vi "SubVI_TeleopIntakeWheels_Teleop.vi"(9 "WheelsShootOut":dbl, 10 "WheelsTakeIn":dbl) -> ()   [LabVIEW 2017]
uses:
  <vilib>/Rock Robotics/WPI/ThirdParty/Phoenix-LabVIEW/Motor Controller/Controls/CTRE_Phoenix_MotorControl_ControlMode.ctl
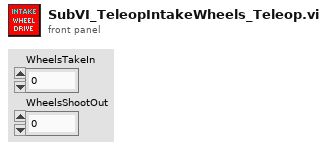
[diagram p1: front panel]
types:
  T1 = typedef "CTRE_Phoenix_MotorControl_ControlMode.ctl" = u16
  T2 = typedef "WPI_MotorControlDeviceRef.ctl" = cluster{"DeviceStatus":errorcluster, "Type":T3, "PWM":cluster{"PWM Channel":T4, "DeadBand":T5}, "CAN":cluster{"Device Number":u8, "SetOutput VI Ref":variant, "GetOutput VI Ref":variant, "Enable VI Ref":variant, "Disable VI Ref":variant, "Data":variant}, "Invert":bool, "DIO PWM":cluster{"PWM \"Enable\" Channel":T4, "DIOChannel":T6, "PWM Rate":dbl}}
  T3 = typedef "WPI_MotorControlType.ctl" = enum16{"PWM", "CAN", "DIO PWM"}
  T4 = typedef "FPGA_DIOPWMChannel.ctl" = enum8{"PWM 0", "PWM 1", "PWM 2", "PWM 3", "PWM 4", "PWM 5", "PWM 6", "PWM 7", "PWM 8", "PWM 9", "PWM MXP 0", "PWM MXP 1", "PWM MXP 2", "PWM MXP 3", "PWM MXP 4", "PWM MXP 5", "PWM MXP 6", "PWM MXP 7", "PWM MXP 8", "PWM MXP 9", "Invalid"}
  T5 = typedef "WPI_PWMDeadband.ctl" = cluster{"Name":string, "maxPositivePwm":i32, "minPositivePwm":i32, "centerPwm":i32, "maxNegativePwm":i32, "minNegativePwm":i32, "angularRange":u16}
  T6 = typedef "FPGA_DIOChannel.ctl" = enum8{"DIO 0", "DIO 1", "DIO 2", "DIO 3", "DIO 4", "DIO 5", "DIO 6", "DIO 7", "DIO 8", "DIO 9", "DIO MXP 0", "DIO MXP 1", "DIO MXP 2", "DIO MXP 3", "DIO MXP 4", "DIO MXP 5", "DIO MXP 6", "DIO MXP 7", "DIO MXP 8", "DIO MXP 9", "DIO MXP 10", "DIO MXP 11", "DIO MXP 12", "DIO MXP 13", "DIO MXP 14", "DIO MXP 15", "SPI Port CS1", "SPI Port CS2", "SPI Port CS3", "SPI Port MISO", "SPI Port MOSI", "Invalid"}
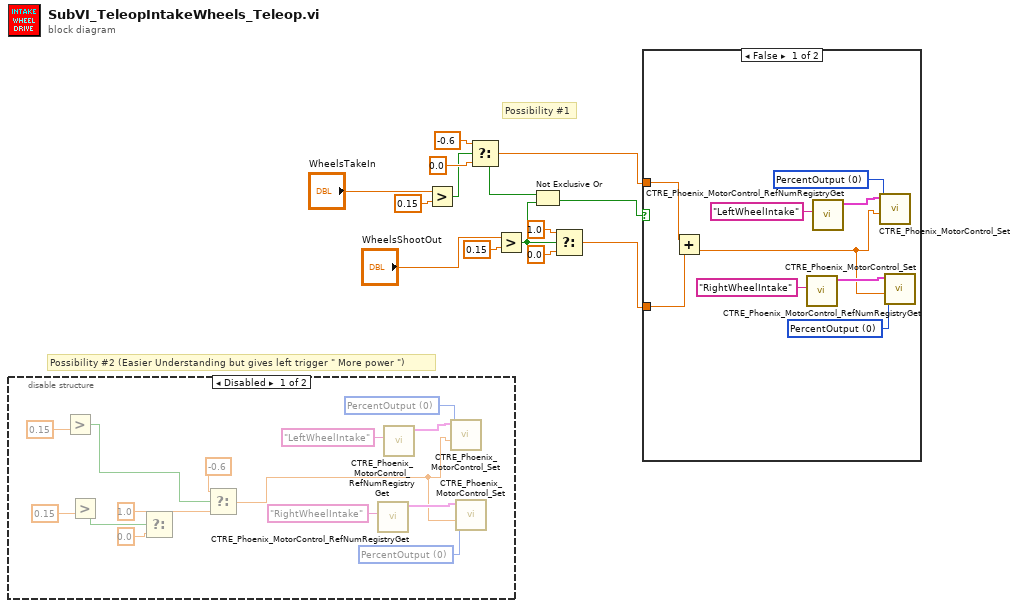
[diagram p0: block diagram]
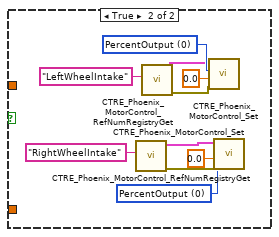
[diagram p3: hidden frame]
diagram:
  # "Possibility #1"
  # "Possibility #2 (Easier Understanding but gives left trigger \" More power \")"
  n1 = disable-structure shown="Disabled" {
    frame Disabled {
      w27 = T1 0 items=["PercentOutput"=0, "Position"=1, "Velocity"=2, "Current"=3, "Follower"=5, "MotionProfile"=6, "MotionMagic"=7, "MotionMagicArc"=8, "MotionProfileArc"=10, "Disabled"=15] ("Control Mode")
      w28 = T1 0 items=["PercentOutput"=0, "Position"=1, "Velocity"=2, "Current"=3, "Follower"=5, "MotionProfile"=6, "MotionMagic"=7, "MotionMagicArc"=8, "MotionProfileArc"=10, "Disabled"=15] ("Control Mode")
      n2 = Greater?(y=0.15) -> (0:w15:bool)  [unwired: 1 in]
      n3 = Greater?(y=0.15) -> (0:w18:bool)  [unwired: 1 in]
      n4 = Select(t=1.0, s=w18, f=0.0) -> (s? t:f=w16:dbl)
      n5 = Select(t=-0.6, s=w15, f=w16) -> (s? t:f=w14:dbl)
      n6 = call <vilib>:"CTRE_Phoenix_MotorControl_RefNumRegistryGet.vi"("refnum name"="RightWheelIntake") -> ("PhoenixMotorControlDevRef"=w25:T2)  [unwired: 9 in, 1 out]
      n7 = call <vilib>:"CTRE_Phoenix_MotorControl_RefNumRegistryGet.vi"("refnum name"="LeftWheelIntake") -> ("PhoenixMotorControlDevRef"=w26:T2)  [unwired: 9 in, 1 out]
      n8 = call <vilib>:"CTRE_Phoenix_MotorControl_Set.vi"("Output"=w14, "Control Mode"=w27, "PhoenixMotorControlDevRef"=w26) -> ()  [unwired: 7 in, 2 out]
      n9 = call <vilib>:"CTRE_Phoenix_MotorControl_Set.vi"("Output"=w14, "Control Mode"=w28, "PhoenixMotorControlDevRef"=w25) -> ()  [unwired: 7 in, 2 out]
    }
    frame Enabled {
    }
  }
  n10 = Greater?(x="WheelsTakeIn", y=0.15) -> (0:w1:bool)
  n11 = Select(t=-0.6, s=w1, f=0.0) -> (s? t:f=w5:dbl)
  n12 = Greater?(x="WheelsShootOut", y=0.15) -> (0:w2:bool)
  n13 = Not Exclusive Or(1:w2, 2:w1) -> (0:w3:bool)
  n14 = Select(t=1.0, s=w2, f=0.0) -> (s? t:f=w4:dbl)
  n15 = case shown="False" w3 {
    tunnel: w5 -> [w31 _]
    tunnel: w4 -> [w30 _]
    frame False {
      w36 = T1 0 items=["PercentOutput"=0, "Position"=1, "Velocity"=2, "Current"=3, "Follower"=5, "MotionProfile"=6, "MotionMagic"=7, "MotionMagicArc"=8, "MotionProfileArc"=10, "Disabled"=15] ("Control Mode")
      w37 = T1 0 items=["PercentOutput"=0, "Position"=1, "Velocity"=2, "Current"=3, "Follower"=5, "MotionProfile"=6, "MotionMagic"=7, "MotionMagicArc"=8, "MotionProfileArc"=10, "Disabled"=15] ("Control Mode")
      n16 = Add(x=w31, y=w30) -> (x+y=w29:dbl)
      n17 = call <vilib>:"CTRE_Phoenix_MotorControl_RefNumRegistryGet.vi"("refnum name"="RightWheelIntake") -> ("PhoenixMotorControlDevRef"=w34:T2)  [unwired: 9 in, 1 out]
      n18 = call <vilib>:"CTRE_Phoenix_MotorControl_RefNumRegistryGet.vi"("refnum name"="LeftWheelIntake") -> ("PhoenixMotorControlDevRef"=w35:T2)  [unwired: 9 in, 1 out]
      n19 = call <vilib>:"CTRE_Phoenix_MotorControl_Set.vi"("Output"=w29, "Control Mode"=w36, "PhoenixMotorControlDevRef"=w35) -> ()  [unwired: 7 in, 2 out]
      n20 = call <vilib>:"CTRE_Phoenix_MotorControl_Set.vi"("Output"=w29, "Control Mode"=w37, "PhoenixMotorControlDevRef"=w34) -> ()  [unwired: 7 in, 2 out]
    }
    frame True {
      w43 = T1 0 items=["PercentOutput"=0, "Position"=1, "Velocity"=2, "Current"=3, "Follower"=5, "MotionProfile"=6, "MotionMagic"=7, "MotionMagicArc"=8, "MotionProfileArc"=10, "Disabled"=15] ("Control Mode")
      w38 = T1 0 items=["PercentOutput"=0, "Position"=1, "Velocity"=2, "Current"=3, "Follower"=5, "MotionProfile"=6, "MotionMagic"=7, "MotionMagicArc"=8, "MotionProfileArc"=10, "Disabled"=15] ("Control Mode")
      n21 = call <vilib>:"CTRE_Phoenix_MotorControl_RefNumRegistryGet.vi"("refnum name"="RightWheelIntake") -> ("error out"=w40:errorcluster, "PhoenixMotorControlDevRef"=w39:T2)  [unwired: 9 in]
      n22 = call <vilib>:"CTRE_Phoenix_MotorControl_RefNumRegistryGet.vi"("refnum name"="LeftWheelIntake") -> ("error out"=w41:errorcluster, "PhoenixMotorControlDevRef"=w42:T2)  [unwired: 9 in]
      n23 = call <vilib>:"CTRE_Phoenix_MotorControl_Set.vi"("error in (no error)"=w41, "Output"=0.0, "Control Mode"=w43, "PhoenixMotorControlDevRef"=w42) -> ()  [unwired: 6 in, 2 out]
      n24 = call <vilib>:"CTRE_Phoenix_MotorControl_Set.vi"("error in (no error)"=w40, "Output"=0.0, "Control Mode"=w38, "PhoenixMotorControlDevRef"=w39) -> ()  [unwired: 6 in, 2 out]
    }
  }
